vi "remove specific errors.vi"(7 "convert to warning? (F)":bool, 8 "error in":errorcluster, 11 "errors to clear":i32[](array[numeric])) -> (0 "error out":errorcluster, 3 "action taken?":bool)   [LabVIEW 2013]
doc: "Converts up to 4 errors into warnings by passing the error code and text of the error received but setting Status of the error to False. This allows the error information to pass without the VI treating the information as an error."
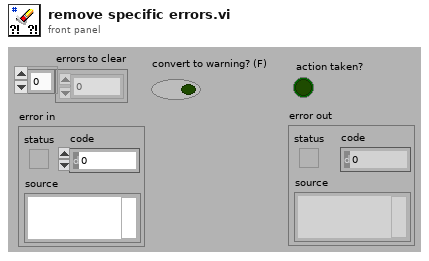
[diagram p1: front panel]
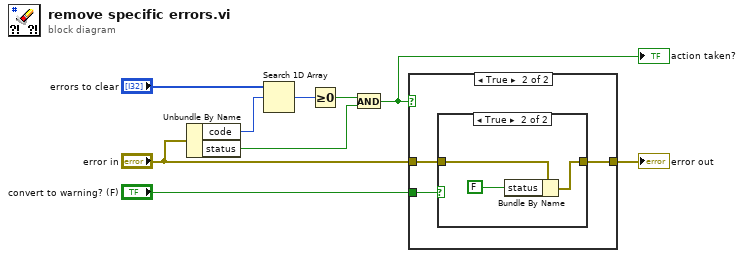
[diagram p0: block diagram]
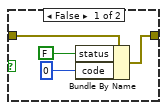
[diagram p3: hidden frame]
diagram:
  n1 = Unbundle By Name("error in") -> ("code"=w3:i32, "status"=w6:bool)
  n2 = Search 1D Array(1D array="errors to clear", element=w3) -> (index of element=w2:i32)  [unwired: 1 in]
  n3 = Greater Or Equal To 0?(x=w2) -> (x >= 0?=w1:bool)
  n4 = And(x=w1, y=w6) -> (x .and. y?=w7:bool)
  "action taken?" <- w7
  n5 = case shown="True" w7 {
    tunnel: "error in" -> [w10 w13]
    tunnel: [w10 w12] -> w8
    tunnel: "convert to warning? (F)" -> [_ w11]
    frame False {
    }
    frame True {
      n6 = case shown="True" w11 {
        tunnel: w13 -> [w17 w20]
        tunnel: [w16 w19] -> w12
        frame False {
          n7 = Bundle By Name(cluster=w17, "status"=FALSE, "code"=0) -> (w16:errorcluster)
        }
        frame True {
          n8 = Bundle By Name(cluster=w20, "status"=FALSE) -> (w19:errorcluster)
        }
      }
    }
  }
  "error out" <- w8
